vi "New Resource Map from Hardware Description.vi"   [LabVIEW 2019, in "Resource Manager.lvlib"]
uses:
  Resource Manager.lvlib
  Constants.vi
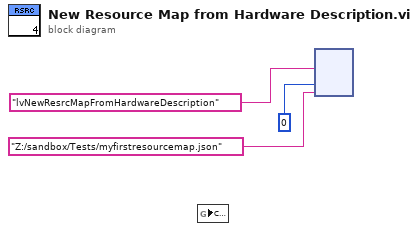
[diagram p0: block diagram]
diagram:
  n1 = global read "Constants.vi" item#-1() -> ()  [unwired: 1 in]
  n2 = node("lvNewResrcMapFromHardwareDescription" ("function name"), 0, "Z:/sandbox/Tests/myfirstresourcemap.json" ("function name")) -> ()  [unwired: 5 in, 4 out]
